vi "CreePosRef.vi"(8 "error in (no error)":errorcluster caption="entrée d'erreur (pas d'erreur)", 10 "Numéro de la référence":u16, 11 "Entrée Variables d'Axes":T1) -> (0 "error out":errorcluster caption="sortie d'erreur", 2 "Position Codeur En Pas":i32)   [LabVIEW 2013]
uses:
  Controls/AdressesVariablesPartagees.ctl
  <vilib>/regexp/Match Regular Expression.xnode
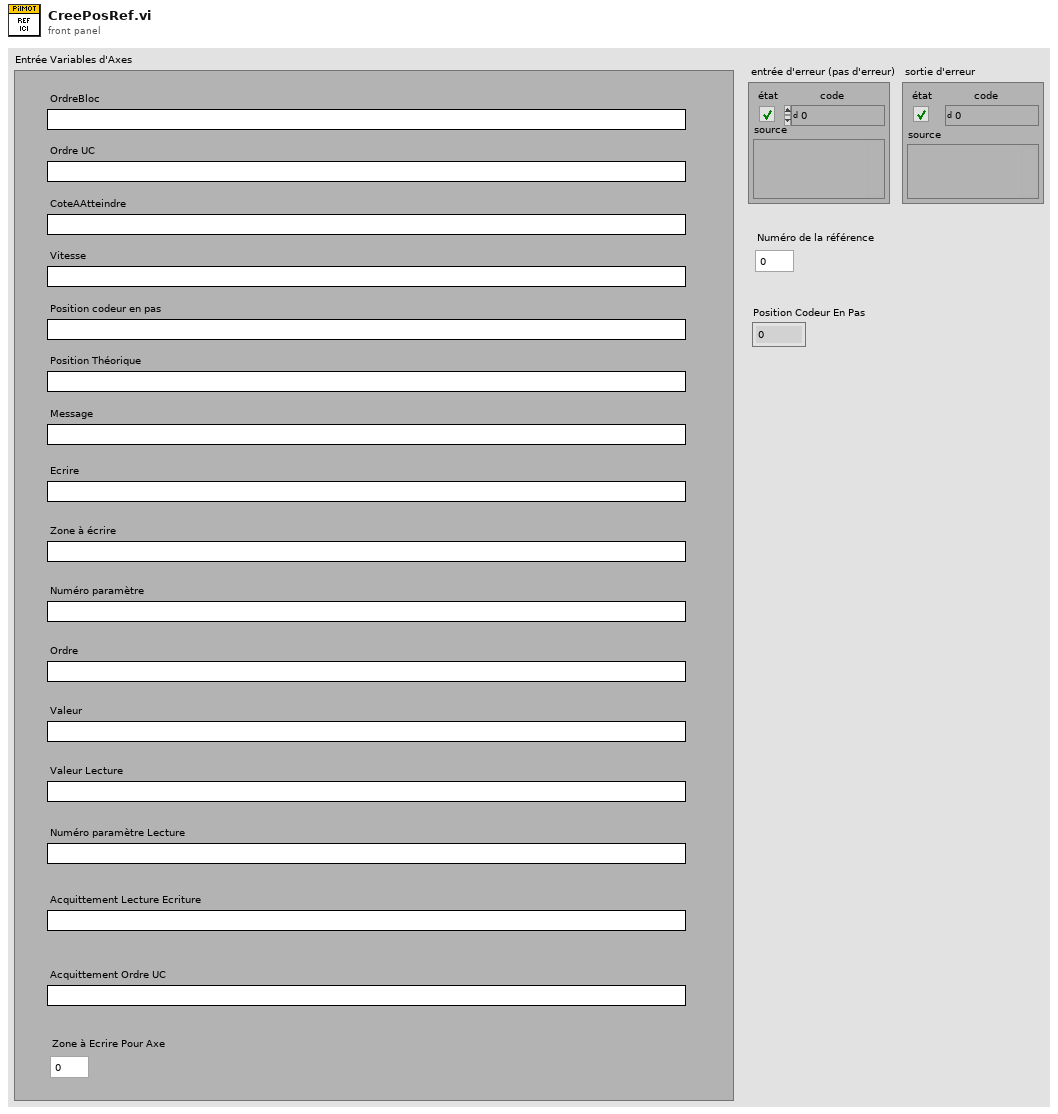
[diagram p1: front panel]
types:
  T1 = typedef "AdressesVariablesPartagees.ctl" = cluster{"OrdreBloc":string, "Ordre UC":string, "CoteAAtteindre":string, "Vitesse":string, "Position codeur en pas":string, "Position Théorique":string, "Message":string, "Ecrire":string, "Zone à écrire":string, "Numéro paramètre":string, "Ordre":string, "Valeur":string, "Valeur Lecture":string, "Numéro paramètre Lecture":string, "Acquittement Lecture Ecriture":string, "Zone à Ecrire Pour Axe ":u16, "Acquittement Ordre UC":string}
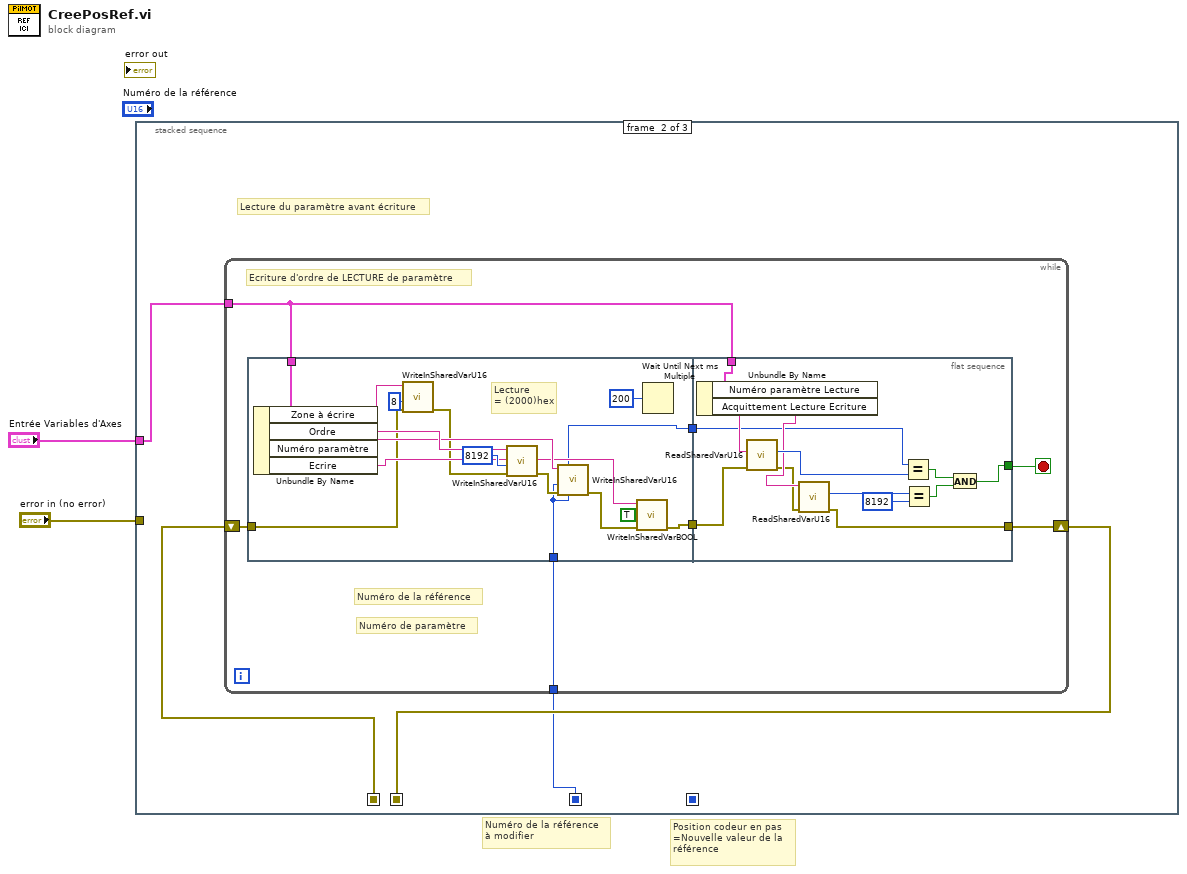
[diagram p0: block diagram]
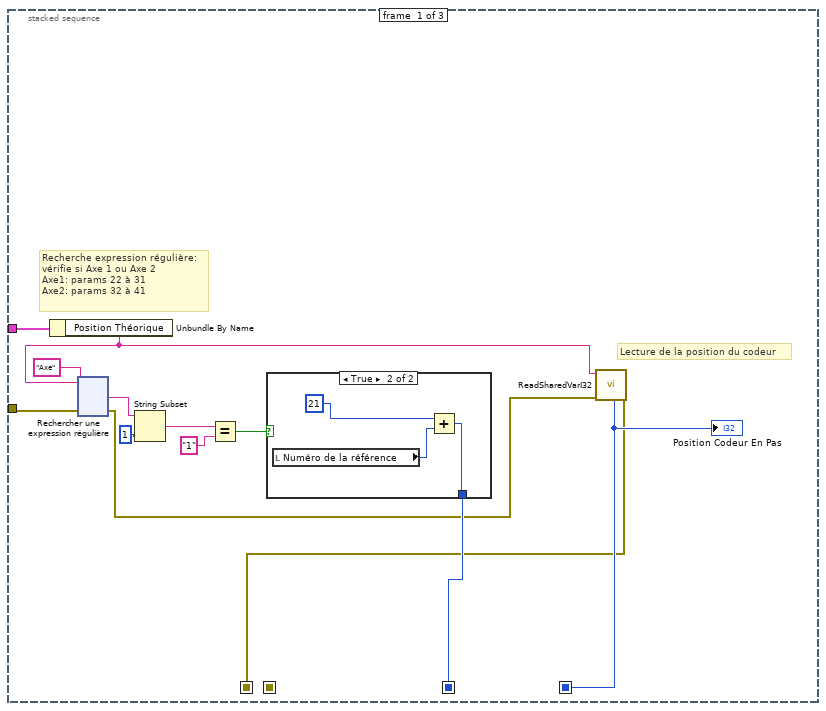
[diagram p2: hidden frame]
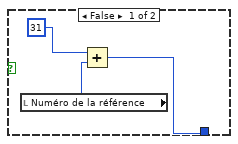
[diagram p3: hidden frame]
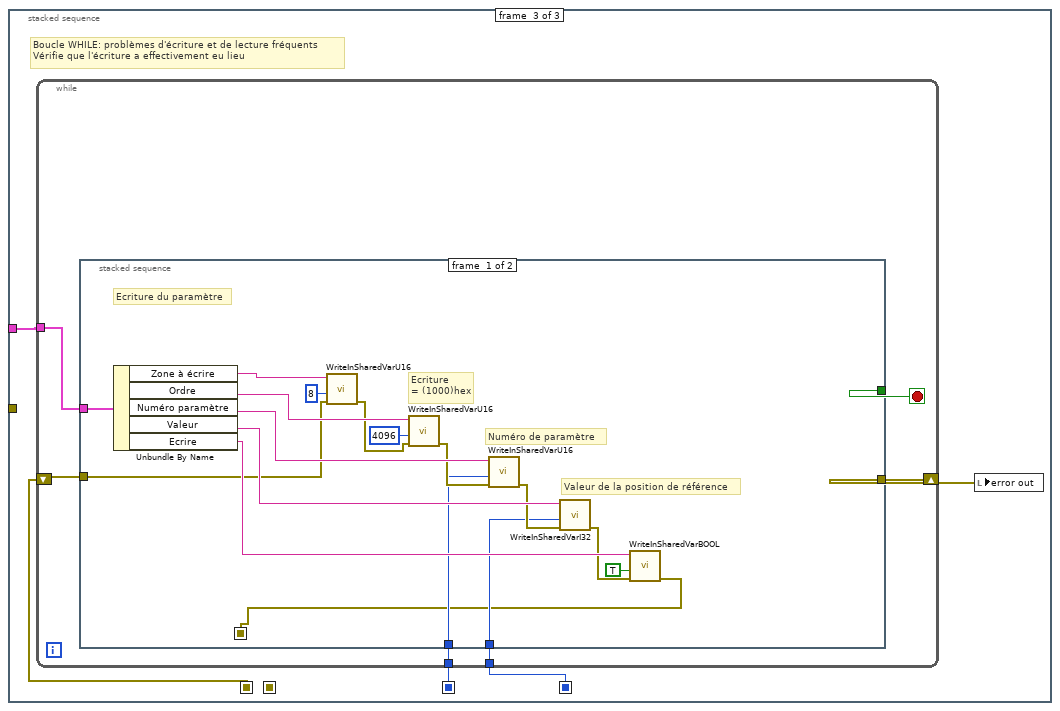
[diagram p4: hidden frame]
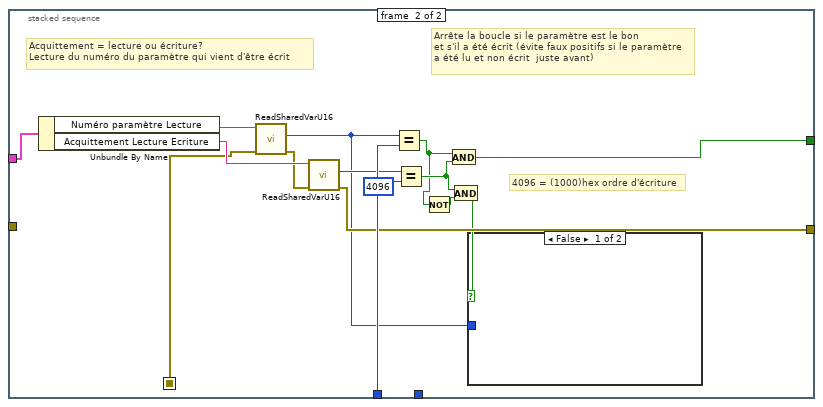
[diagram p5: hidden frame]
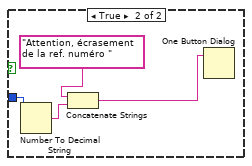
[diagram p6: hidden frame]
diagram:
  # "Position codeur en pas\n=Nouvelle valeur de la \nréférence"
  # "Numéro de la référence\nà modifier"
  n1 = stacked-sequence {
    seq-local: [w3 _ _] -> [_ w139 w176]
    seq-local: [w8 _ _] -> [_ w136 w178]
    seq-local: [w7 _ _] -> [_ _ w177]
    seq-local: [_ w137 _] -> [_ _ _]
    tunnel: "Entrée Variables d'Axes" -> [w15 w138 w179]
    tunnel: "error in (no error)" -> [w6 _ _]
    frame #0 {
      # "Lecture de la position du codeur"
      # "Recherche expression régulière:\nvérifie si Axe 1 ou Axe 2\nAxe1: params 22 à 31\nAxe2: params 32 à 41"
      n2 = Unbundle By Name(w15) -> ("Position Théorique"=w4:string)
      n3 = xnode "Rechercher une expression régulière"("chaîne en entrée"=w4, "expression régulière"="Axe", "entrée d'erreur"=w6) -> ("après la correspondance"=w13:string, "sortie d'erreur"=w5:errorcluster)  [unwired: 3 in, 3 out]
      n4 = String Subset(string=w13, length (rest)=1 ("longueur (reste)")) -> (substring=w10:string)  [unwired: 1 in]
      n5 = Equal?(x=w10, y="1") -> (x = y?=w9:bool)
      n6 = case shown="True" w9 {
        tunnel: [w16 w19] -> w8
        frame False {
          n7 = local read "Numéro de la référence"() -> (w17:u16)
          n8 = Add(x=u16 31 ("Offset Paramètre"), y=w17) -> (x+y=w16:u16)
        }
        frame True {
          n9 = local read "Numéro de la référence"() -> (w20:u16)
          n10 = Add(x=u16 21 ("Offset Paramètre"), y=w20) -> (x+y=w19:u16)
        }
      }
      n11 = call "ReadSharedVarI32.vi"("entrée d'erreur (pas d'erreur)"=w5, "refnum de variable partagée en entrée"=w4) -> ("sortie d'erreur"=w3:errorcluster, "données en sortie"=w7:i32)  [unwired: 8 in]
      "Position Codeur En Pas" <- w7
    }
    frame #1 {
      # "Lecture du paramètre avant écriture"
      n12 = while {
        tunnel: w138 -> [w144]
        shift-right: [w143] -> w137
        shift-left: w139 -> [w142]
        tunnel: w136 -> [w140]
        stop <- w145 stop-if-true
        # "Numéro de la référence"
        # "Ecriture d'ordre de LECTURE de paramètre"
        # "Numéro de paramètre"
        n13 = flat-sequence {
          tunnel: w144 -> [w161]
          tunnel: [w154] -> w146
          tunnel: w142 -> [w149]
          tunnel: [w148] -> w141
          tunnel: w140 -> [w148]
          tunnel: [w166] -> w143
          tunnel: w146 -> [w172]
          tunnel: [w163] -> w145
          tunnel: w144 -> [w174]
          tunnel: w141 -> [w162]
          frame #0 {
            # "Lecture \n= (2000)hex"
            n14 = Unbundle By Name(w161) -> ("Zone à écrire"=w153:string, "Ordre"=w160:string, "Numéro paramètre"=w158:string, "Ecrire"=w156:string)
            n15 = call "WriteInSharedVarU16.vi"("entrée d'erreur (pas d'erreur)"=w149, "données en entrée"=u16 8, "refnum de variable partagée en entrée"=w153) -> ("sortie d'erreur"=w151:errorcluster)  [unwired: 8 in]
            n16 = call "WriteInSharedVarU16.vi"("entrée d'erreur (pas d'erreur)"=w151, "données en entrée"=u16 8192, "refnum de variable partagée en entrée"=w160) -> ("sortie d'erreur"=w157:errorcluster)  [unwired: 8 in]
            n17 = call "WriteInSharedVarU16.vi"("entrée d'erreur (pas d'erreur)"=w157, "données en entrée"=w148, "refnum de variable partagée en entrée"=w158) -> ("sortie d'erreur"=w155:errorcluster)  [unwired: 8 in]
            n18 = call "WriteInSharedVarBOOL.vi"("entrée d'erreur (pas d'erreur)"=w155, "données en entrée"=TRUE, "refnum de variable partagée en entrée"=w156) -> ("sortie d'erreur"=w154:errorcluster)  [unwired: 8 in]
            n19 = Wait Until Next ms Multiple(millisecond multiple=u32 200 ("n millisecondes")) -> ()  [unwired: 1 out]
          }
          frame #1 {
            n20 = Unbundle By Name(w174) -> ("Numéro paramètre Lecture"=w173:string, "Acquittement Lecture Ecriture"=w170:string)
            n21 = call "ReadSharedVarU16.vi"("entrée d'erreur (pas d'erreur)"=w172, "refnum de variable partagée en entrée"=w173) -> ("sortie d'erreur"=w167:errorcluster, "données en sortie"=w171:u16)  [unwired: 8 in]
            n22 = call "ReadSharedVarU16.vi"("entrée d'erreur (pas d'erreur)"=w167, "refnum de variable partagée en entrée"=w170) -> ("sortie d'erreur"=w166:errorcluster, "données en sortie"=w169:u16)  [unwired: 8 in]
            n23 = Equal?(x=w162, y=w171) -> (x = y?=w165:bool)
            n24 = Equal?(x=w169, y=u16 8192) -> (x = y?=w164:bool)
            n25 = And(x=w165, y=w164) -> (x .and. y?=w163:bool)
          }
        }
      }
    }
    frame #2 {
      # "Boucle WHILE: problèmes d'écriture et de lecture fréquents\nVérifie que l'écriture a effectivement eu lieu"
      n26 = while {
        tunnel: w179 -> [w185]
        tunnel: w178 -> [w184]
        tunnel: w177 -> [w183]
        shift-right: [w180] -> w175
        shift-left: w176 -> [w182]
        stop <- w181 stop-if-true
        n27 = stacked-sequence {
          seq-local: [w186 _] -> [_ w203]
          tunnel: w185 -> [w202 w217]
          tunnel: w184 -> [w190 w215]
          tunnel: w183 -> [w189 _]
          tunnel: w182 -> [w187 _]
          tunnel: [_ w210] -> w181
          tunnel: [_ w209] -> w180
          frame #0 {
            # "Ecriture du paramètre"
            # "Valeur de la position de référence"
            # "Numéro de paramètre"
            # "Ecriture \n= (1000)hex"
            n28 = Unbundle By Name(w202) -> ("Zone à écrire"=w201:string, "Ordre"=w199:string, "Numéro paramètre"=w197:string, "Valeur"=w196:string, "Ecrire"=w195:string)
            n29 = call "WriteInSharedVarU16.vi"("entrée d'erreur (pas d'erreur)"=w187, "données en entrée"=u16 8, "refnum de variable partagée en entrée"=w201) -> ("sortie d'erreur"=w194:errorcluster)  [unwired: 8 in]
            n30 = call "WriteInSharedVarU16.vi"("entrée d'erreur (pas d'erreur)"=w194, "données en entrée"=u16 4096, "refnum de variable partagée en entrée"=w199) -> ("sortie d'erreur"=w193:errorcluster)  [unwired: 8 in]
            n31 = call "WriteInSharedVarU16.vi"("entrée d'erreur (pas d'erreur)"=w193, "données en entrée"=w190, "refnum de variable partagée en entrée"=w197) -> ("sortie d'erreur"=w192:errorcluster)  [unwired: 8 in]
            n32 = call "WriteInSharedVarI32.vi"("entrée d'erreur (pas d'erreur)"=w192, "données en entrée"=w189, "refnum de variable partagée en entrée"=w196) -> ("sortie d'erreur"=w191:errorcluster)  [unwired: 8 in]
            n33 = call "WriteInSharedVarBOOL.vi"("entrée d'erreur (pas d'erreur)"=w191, "données en entrée"=TRUE, "refnum de variable partagée en entrée"=w195) -> ("sortie d'erreur"=w186:errorcluster)  [unwired: 8 in]
          }
          frame #1 {
            # "4096 = (1000)hex ordre d'écriture"
            # "Arrête la boucle si le paramètre est le bon\net s'il a été écrit (évite faux positifs si le paramètre\na été lu et non écrit  juste avant)"
            # "Acquittement = lecture ou écriture? \nLecture du numéro du paramètre qui vient d'être écrit"
            n34 = Unbundle By Name(w217) -> ("Numéro paramètre Lecture"=w216:string, "Acquittement Lecture Ecriture"=w214:string)
            n35 = call "ReadSharedVarU16.vi"("entrée d'erreur (pas d'erreur)"=w203, "refnum de variable partagée en entrée"=w216) -> ("sortie d'erreur"=w213:errorcluster, "données en sortie"=w204:u16)  [unwired: 8 in]
            n36 = call "ReadSharedVarU16.vi"("entrée d'erreur (pas d'erreur)"=w213, "refnum de variable partagée en entrée"=w214) -> ("sortie d'erreur"=w209:errorcluster, "données en sortie"=w212:u16)  [unwired: 8 in]
            n37 = Equal?(x=w204, y=w215) -> (x = y?=w206:bool)
            n38 = Equal?(x=w212, y=u16 4096) -> (x = y?=w208:bool)
            n39 = Not(x=w206) -> (.not. x?=w207:bool)
            n40 = And(x=w206, y=w208) -> (x .and. y?=w210:bool)
            n41 = And(x=w208, y=w207) -> (x .and. y?=w205:bool)
            n42 = case shown="False" w205 {
              tunnel: w204 -> [_ w221]
              frame False {
              }
              frame True {
                n43 = Number To Decimal String(number=w221) -> (decimal integer string=w220:string)  [unwired: 1 in]
                n44 = Concatenate Strings("Attention, écrasement de la ref. numéro " ("message"), w220) -> (w218:string)
                n45 = One Button Dialog(message=w218) -> ()  [unwired: 1 in, 1 out]
              }
            }
          }
        }
      }
      n46 = local write "error out"(w175) -> ()
    }
  }
